vi "CANTest.vi"(0 "设备类型":u32(ring)=3 items=["PCI5121"=1, "PCI9810"=2, "USBCAN1"=3, "USBCAN2"=4, "PCI9820"=5, "PCI5110"=7, "PC104CAN"=11, "CANETUDP"=12, "PCI9840B"=14, "PC104C2"=15, "PCI9820I"=16, "CANETTCP"=17, "PCIE9221"=24, "PCI5010U"=19, "USBCAN_E_U"=20, "USBCAN_2E_U"=21, "PCI5020U"=22], 1 "数据输入":string="0011223344556677", 2 "Baud":u32(ring)=11 caption="波特率" items=["5Kbps", "10Kbps", "20Kbps", "40Kbps", "50Kbps", "80Kbps", "100Kbps", "125Kbps", "200Kbps", "250Kbps", "400Kbps", "500Kbps", "666Kbps", "800Kbps", "1000Kbps"], 5 "DevIndex":u32, 7 "CANInd":u32, 9 "ID":string="666;667", 11 "error in":errorcluster caption="错误输入", 12 "滤波":bool, 13 "发送类型":u8(ring) items=["正常发送", "单次发送", "自发自收", "单次自发自收"]) -> (4 "Result":bool, 8 "VCI_CAN_OBJ_RN":T1(array[cluster]) {"Byte7" format="%02x"; "Byte6" format="%02x"; "Byte5" format="%02x"; "Byte4" format="%02x"; "Byte3" format="%02x"; "Byte2" format="%02x"; "Byte1" format="%02x"; "Byte0" format="%02x"; "ID" format="%.0x"}, 15 "error out":errorcluster caption="错误输出")   [LabVIEW 2013]
uses:
  ControlCAN.dll
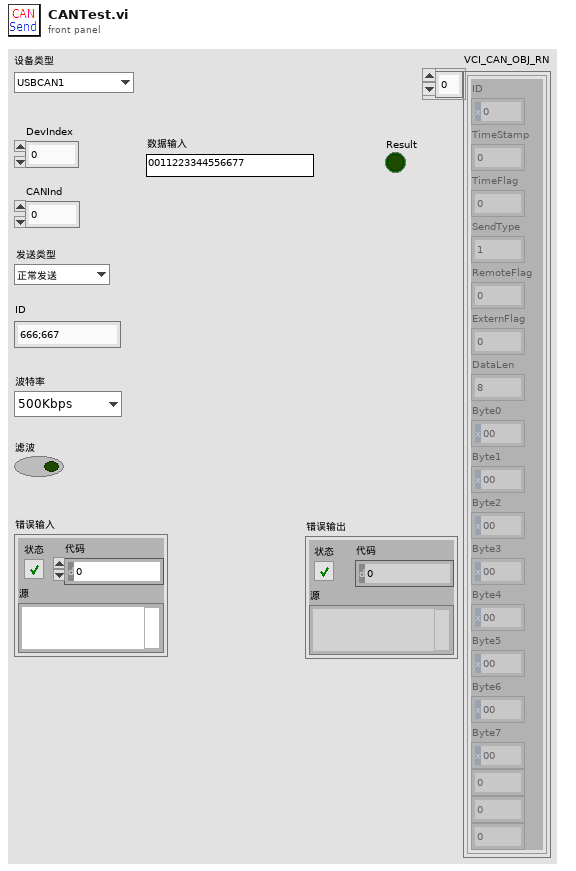
[diagram p1: front panel]
types:
  T1 = cluster{"ID":u32, "TimeStamp":u32, "TimeFlag":u8, "SendType":u8, "RemoteFlag":u8, "ExternFlag":u8, "DataLen":u8, "Byte0":u8, "Byte1":u8, "Byte2":u8, "Byte3":u8, "Byte4":u8, "Byte5":u8, "Byte6":u8, "Byte7":u8, u8, u8, u8}[]
  T2 = cluster{"ID":u32, "TimeStamp":u32, "TimeFlag":u8, "SendType":u8, "RemoteFlag":u8, "ExternFlag":u8, "DataLen":u8, u8, u8, u8, u8, u8, u8, u8, u8, u8, u8, u8}
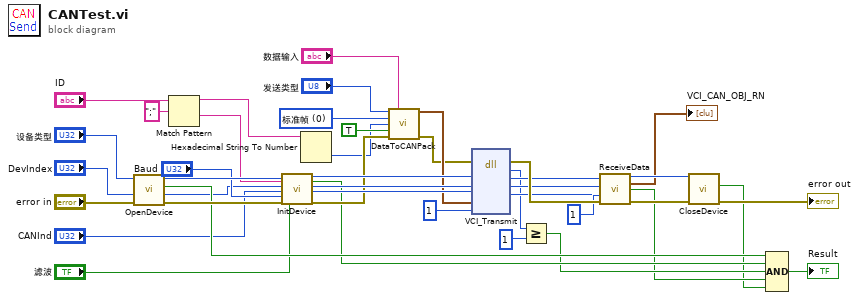
[diagram p0: block diagram]
diagram:
  w42 = u8 0 items=["标准帧", "扩展帧"] ("帧类型")
  n1 = call "OpenDevice.vi"("错误输入（无错误）"="error in", "DevIndex"="DevIndex", "设备类型"="设备类型") -> ("错误输出"=w35:errorcluster, "DevInd"=w7:u32, "Result"=w14:bool, "DevType"=w37:u32)  [unwired: 5 in]
  n2 = Match Pattern(string="ID", regular expression=";" ("正则表达式")) -> (before substring=w2:string, after substring=w1:string)  [unwired: 1 in, 2 out]
  n3 = call "InitDevice.vi"("设备类型"=w37, "ID(Hex 高位有效)"=w1, "DeviceInd"=w7, "CANInd"="CANInd", "Baud"="Baud", "错误输入（无错误）"=w35, "滤波"="滤波") -> ("DeviceType"=w33:u32, "Result"=w13:bool, "DeviceIndex"=w31:u32, "CANIndex"=w30:u32, "错误输出"=w28:errorcluster)  [unwired: 8 in]
  n4 = Hexadecimal String To Number(string=w2) -> (number=w8:u32)  [unwired: 2 in, 1 out]
  n5 = call "DataToCANPack.vi"("发送类型"="发送类型", "数据输入"="数据输入", "帧类型"=w42, "ID"=w8, "启用"=TRUE, "error in"=w28) -> ("VCI_CAN_OBJT"=w29:T2, "error out"=w27:errorcluster)  [unwired: 8 in]
  n6 = dll-call lib="PTH1`abs E桌面休眠电流方案休眠电流源码20190314\nInstrumentCANControlCAN.dll" fn="VCI_Transmit" label="VCI_T"(error in=w27, "DeviceType"=w33, "DeviceInd"=w31, "CANInd"=w30, "pSend"=w29, "Len"=u32 1) -> (error out=w24:errorcluster, "return type"=w16:u32, "DeviceType"=w19:u32, "DeviceInd"=w18:u32, "CANInd"=w17:u32)  [unwired: 3 in, 2 out]
  n7 = Greater Or Equal?(x=w16, y=u32 1 ("arraylen")) -> (x >= y?=w12:bool)
  n8 = call "ReceiveData.vi"("设备类型"=w19, "索引号"=w18, "CAN通道"=w17, "arraylen"=u32 1, "错误输入"=w24) -> ("DeviceType"=w21:u32, "VCI_CAN_OBJ_RN"=→"VCI_CAN_OBJ_RN":T1, "Result"=w11:bool, "错误输出"=w23:errorcluster)  [unwired: 6 in, 1 out]
  n9 = call "CloseDevice.vi"("错误输入（无错误）"=w23, "设备类型"=w21) -> ("错误输出"=→"error out":errorcluster, "Result"=w10:bool)  [unwired: 8 in]
  n10 = Compound Arithmetic op=AND(w14, w13, w12, w11, w10) -> (→"Result":bool)
